vi "HumanSwerveDrive.vi"(8 "Enable Field Oriented Drive":bool, 9 "Rotation":dbl, 10 "Y":dbl, 11 "X":dbl) -> (1 "A":dbl, 2 "Y":dbl, 3 "X":dbl)   [LabVIEW 2023]
uses:
  <vilib>/Rock Robotics/WPI/ThirdParty/JAS_Junk/TrajLib/Trajectory_Library.lvlib
panel:
  # "we switched these, hopefully it is right"
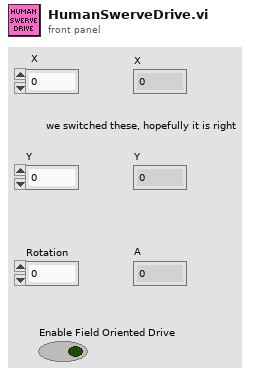
[diagram p1: front panel]
types:
  T1 = typedef "Trajectory_Library.lvlib/ROTATION2D.ctl" = cluster{"VALUE":dbl, "COS":dbl, "SIN":dbl}
  T2 = typedef "Trajectory_Library.lvlib/TRANSLATION2D.ctl" = cluster{"X":dbl, "Y":dbl}
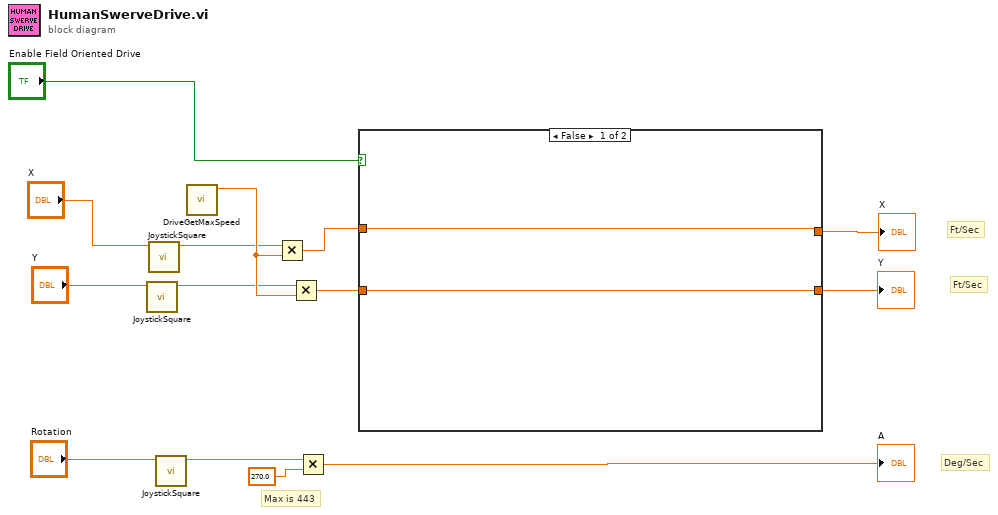
[diagram p0: block diagram]
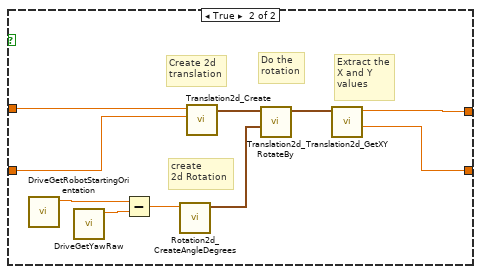
[diagram p2: hidden frame]
diagram:
  # "Deg/Sec"
  # "Ft/Sec"
  # "Ft/Sec"
  # "Max is 443"
  n1 = call "JoystickSquare.vi"("JoyStickInput"="Y") -> ("SquaredOutput"=w3:dbl)  [unwired: 10 in]
  n2 = call "JoystickSquare.vi"("JoyStickInput"="X") -> ("SquaredOutput"=w5:dbl)  [unwired: 10 in]
  n3 = call "JoystickSquare.vi"("JoyStickInput"="Rotation") -> ("SquaredOutput"=w1:dbl)  [unwired: 10 in]
  n4 = call "DriveGetMaxSpeed.vi"() -> ("Max Speed (ft/sec)"=w7:dbl)  [unwired: 11 in]
  n5 = Multiply(x=w5, y=w7) -> (x*y=w13:dbl)
  n6 = Multiply(x=w3, y=w7) -> (x*y=w14:dbl)
  n7 = Multiply(x=w1, y=270.0) -> (x*y=→"A":dbl)
  n8 = case shown="False" "Enable Field Oriented Drive" {
    tunnel: w14 -> [w15 w22]
    tunnel: w13 -> [w16 w21]
    tunnel: [w16 w18] -> w10
    tunnel: [w15 w17] -> w9
    frame False {
    }
    frame True {
      # "Extract the\nX and Y \nvalues"
      # "Do the \nrotation"
      # "Create 2d\ntranslation"
      # "create\n2d Rotation"
      n9 = call "DriveGetRobotStartingOrientation.vi"() -> ("RobotInitalOrientationDeg"=w20:dbl)  [unwired: 11 in]
      n10 = call "DriveGetYawRaw.vi"() -> ("YawRaw"=w19:dbl)  [unwired: 11 in]
      n11 = Subtract(x=w20, y=w19) -> (x-y=w26:dbl)
      n12 = call <vilib>:"Rotation2d_CreateAngleDegrees.vi"("Angle_Degrees"=w26) -> ("ROTATION"=w24:T1)  [unwired: 10 in]
      n13 = call <vilib>:"Translation2d_Create.vi"("Y"=w22, "X"=w21) -> ("TRANSLATION"=w23:T2)  [unwired: 9 in]
      n14 = call <vilib>:"Translation2d_RotateBy.vi"("other Rotation"=w24, "In Translation"=w23) -> ("Out Translation"=w25:T2)  [unwired: 9 in]
      n15 = call <vilib>:"Translation2d_GetXY.vi"("In Translation"=w25) -> ("Y"=w17:dbl, "X"=w18:dbl)  [unwired: 9 in]
    }
  }
  "Y" <- w9
  "X" <- w10
